vi "Initialize Sessions with Retry.vi"(6 "initialize and close session behavior":T1, 7 "require single session":bool, 8 "error in":errorcluster, 10 "instrument":refnum<class "ISession Factory.lvclass">, 11 "session reservation in":refnum<class "Session Reservation.lvclass">) -> (0 "error out":errorcluster, 1 "channel lists":string[](array[string]), 2 "sessions":variant[](array[variant]), 3 "session reservation out":refnum<class "Session Reservation.lvclass">)   [LabVIEW 2020, in "NI Session Management V1 Client.lvlib" / "Session Reservation.lvclass"]
uses:
  Session Reservation.lvclass
  Sessions/Instrument/ISession Factory/ISession Factory.lvclass
  Initialize and Close Session Behavior.ctl
  Discovery V1/TypeDefs/Service Location FGV Action.ctl
  gRPC/Generated APIs/ni/measurementlink/discovery/v1/RPC Messages/ni_measurementlink_discovery_v1_ResolveServiceRequest.ctl
  Discovery V1/NI Discovery V1 Client.lvlib
  gRPC/Generated APIs/ni/measurementlink/discovery/v1/ni.measurementlink.discovery.v1.api.lvlib
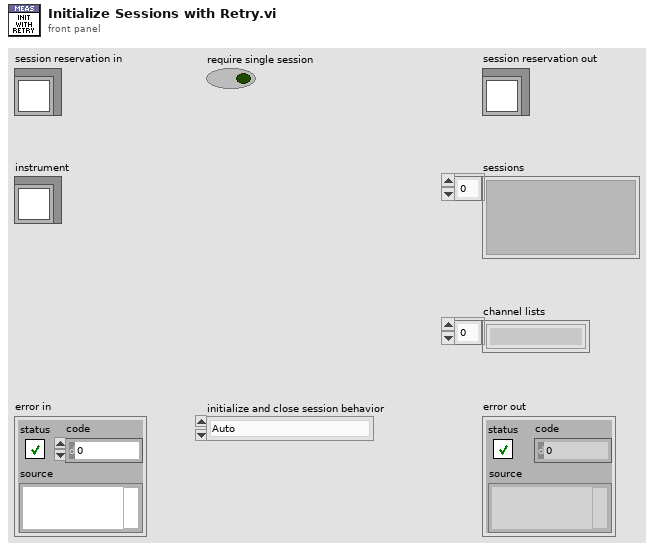
[diagram p1: front panel]
types:
  T1 = typedef "NI Session Management V1 Client.lvlib/Session Reservation.lvclass/Initialize and Close Session Behavior.ctl" = enum16{"Auto", "Initialize and Close", "Attach and Detach", "Initialize and Detach", "Attach and Close"}
  T2 = typedef "ni.measurementlink.discovery.v1.api.lvlib/ni_measurementlink_discovery_v1_ResolveServiceRequest.ctl" = cluster{"provided_interface":string, "service_class":string}
  T3 = typedef "NI Discovery V1 Client.lvlib/Service Location FGV Action.ctl" = enum16{"Get Service Location", "Reresolve Service Location"}
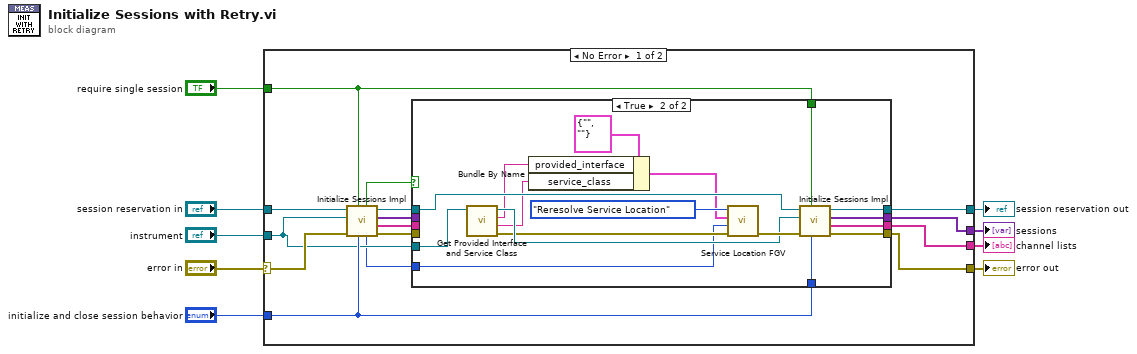
[diagram p0: block diagram]
diagram:
  n1 = case shown="No Error" "error in" {
    selector: "error in" -> [w23 w47]
    tunnel: [w21 w47] -> w8
    tunnel: [w15 w46] -> w6
    tunnel: "session reservation in" -> [w24 w46]
    tunnel: "instrument" -> [w12 _]
    tunnel: [w19 _] -> w3
    tunnel: [w17 _] -> w4
    tunnel: "require single session" -> [w13 _]
    tunnel: "initialize and close session behavior" -> [w14 _]
    frame No Error {
      n2 = call "Initialize Sessions Impl.vi"("initialize and close session behavior"=w14, "require single session"=w13, "error in"=w23, "instrument"=w12, "session reservation in"=w24) -> ("error out"=w22:errorcluster, "channel lists"=w18:string[], "sessions"=w20:variant[], "session reservation out"=w16:refnum<class "Session Reservation.lvclass">, "location unique id"=w11:u64, "retry"=w10:bool)  [unwired: 1 in]
      n3 = case shown="True" w10 {
        tunnel: w22 -> [w28 _]
        tunnel: [w28 w41] -> w21
        tunnel: w20 -> [w27 _]
        tunnel: [w27 w44] -> w19
        tunnel: w18 -> [w26 _]
        tunnel: [w26 w45] -> w17
        tunnel: w16 -> [w25 w43]
        tunnel: [w25 w40] -> w15
        tunnel: w14 -> [_ w42]
        tunnel: w13 -> [_ w39]
        tunnel: w12 -> [_ w36]
        tunnel: w11 -> [_ w29]
        frame False {
        }
        frame True {
          n4 = call "Get Provided Interface and Service Class.vi"("instrument in"=w36) -> ("error out"=w34:errorcluster, "service class"=w31:string, "provided interface"=w32:string, "instrument out"=w35:refnum<class "ISession Factory.lvclass">)  [unwired: 6 in, 1 out]
          n5 = Bundle By Name(cluster=T2 {"provided_interface"="", "service_class"=""} ("resolve service request"), "provided_interface"=w32, "service_class"=w31) -> (w30:T2)
          n6 = call "Service Location FGV.vi"("error in"=w34, "location unique id in"=w29, "resolve service request"=w30, "action"=Service_Location_FGV_Action."Reresolve Service Location") -> ("error out"=w37:errorcluster)  [unwired: 5 in, 2 out]
          n7 = call "Initialize Sessions Impl.vi"("initialize and close session behavior"=w42, "require single session"=w39, "error in"=w37, "instrument"=w35, "session reservation in"=w43) -> ("error out"=w41:errorcluster, "channel lists"=w45:string[], "sessions"=w44:variant[], "session reservation out"=w40:refnum<class "Session Reservation.lvclass">)  [unwired: 1 in, 2 out]
        }
      }
    }
    frame Error {
    }
  }
  "error out" <- w8
  "session reservation out" <- w6
  "channel lists" <- w4
  "sessions" <- w3
